vi "Get Angle.vi"(8 "error in":errorcluster, 10 "array":dbl[](array[numeric]), 11 "input cluster":T1) -> (0 "error out":errorcluster, 3 "output cluster":T1)   [LabVIEW 2021, in "Component Tray.lvclass"]
uses:
  Component Tray.lvclass
  Find Component.ctl
  Controller/Camera/Machine Vision.ctl
  Controller/Camera/Camera.lvclass
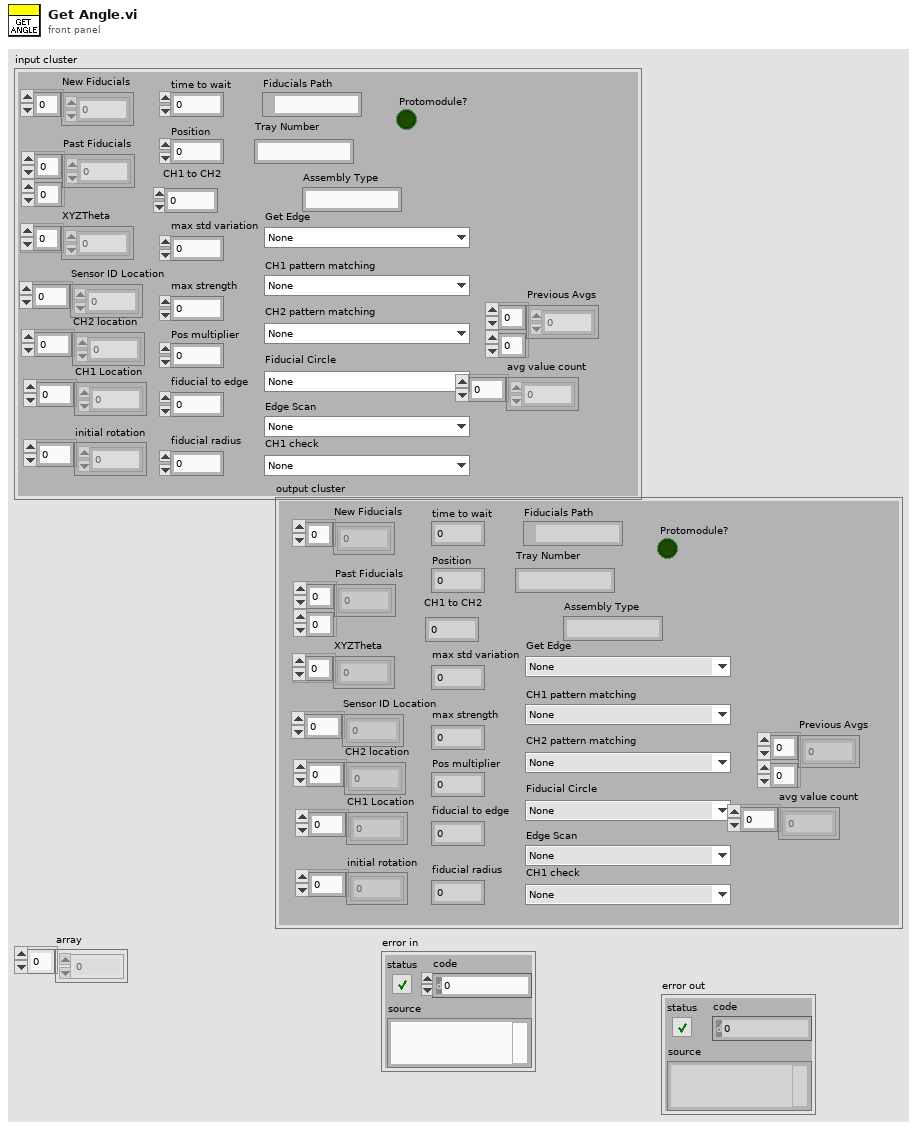
[diagram p1: front panel]
types:
  T1 = typedef "Component Tray.lvclass/Find Component.ctl" = cluster{"New Fiducials":dbl[], "Past Fiducials":dbl[][], "XYZTheta":dbl[], "Fiducials Path":path, "Position":i32, "CH1 Location":dbl[], "Sensor ID Location":dbl[], "initial rotation":dbl[], "CH2 location":dbl[], "max std variation":dbl, "max strength":dbl, "CH2 pattern matching":T2, "Fiducial Circle":T2, "Get Edge":T2, "Pos multiplier":dbl, "time to wait":u32, "fiducial to edge":dbl, "Protomodule?":bool, "Assembly Type":string, "CH1 to CH2":dbl, "Tray Number":string, "fiducial radius":dbl, "4 fiducials?":bool, "CH1 check":T2, "Edge Scan":T2, "CH1 pattern matching":T2, "Sensor Thickness":dbl, "Previous Avgs":dbl[][], "avg value count":dbl[]}
  T2 = typedef "Camera.lvclass/Machine Vision.ctl" = enum16{"None", "Assembly Tray Circle", "Assembly Tray Fiducial", "Partial Hexaboard", "sensor edge init", "HB edge init", "sensor edge pos1", "sensor edge pos2", "HB edge pos1", "HB edge pos2", "Sensor CH1-2", "HB CH1", "HB CH2", "V3 Sensor Circle", "Hexaboard Circle", "sensor CH1 check", "HB CH1 check ", "sensor ID"}
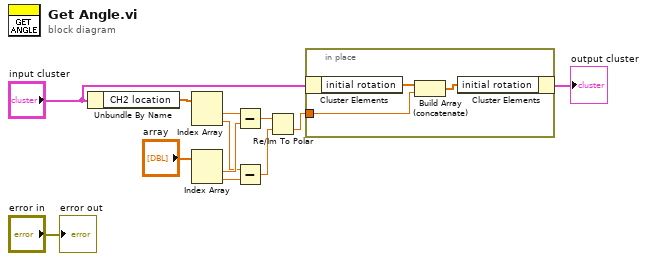
[diagram p0: block diagram]
diagram:
  n1 = Unbundle By Name("input cluster") -> ("CH2 location"=w10:dbl[])
  n2 = Index Array(array=w10) -> (element #1=w8:dbl, element #2=w6:dbl)  [unwired: 2 in]
  n3 = Index Array(array="array") -> (element #1=w7:dbl, element #2=w5:dbl)  [unwired: 2 in]
  n4 = Subtract(x=w8, y=w7) -> (x-y=w4:dbl)
  n5 = Subtract(x=w6, y=w5) -> (x-y=w3:dbl)
  n6 = Re/Im To Polar(2:w3, 3:w4) -> (0:w2:dbl)  [unwired: 1 out]
  n7 = in-place {
    in-place-border: w2 -> [w13]
    n8 = in-place-cluster #1("input cluster") -> ("initial rotation"=w15:dbl[])
    n9 = Build Array (concatenate)(w15, w13) -> (w14:dbl[])
    n10 = in-place-cluster #1("initial rotation"=w14) -> (→"output cluster":T1)
  }
  "error out" <- "error in"
